vi "Teleop.vi"(10 "Match Info":T1={"Autonomous Elapsed Seconds"=0.0, "TeleOp Elapsed Seconds"=0.0, "Disabled Elapsed Seconds"=0.0, "Visited Autonomous"=FALSE, "Visited TeleOp"=FALSE, "Visited Disabled"=FALSE, "Autonomous Settings"={"Autonomous Style"=enum."Independent", "VI Refnum"=refnum}}, 11 "Call Context":T2) -> ()   [LabVIEW 2019]
doc: "This VI is called for each TeleOp packet received from the DS where the robot is not disabled. It is often used to read from the joysticks and update I/O or to update setpoints for timed control loops. It should complete and return within 20 milliseconds or it may miss DS packets."
uses:
  <vilib>/Rock Robotics/WPI/DriverStation/WPI_DriverStationDerivedRobotMode.ctl
  <vilib>/Rock Robotics/WPI/DriverStation/WPI_DriverStationMatch Info.ctl
  <vilib>/Rock Robotics/WPI/Utilities/WPI_GetSetVariantRefNum.vi
  Robot Global Data.vi
  fe9523e3-5247-4d02-ac38-c1c90a242367.vi
  0c9b3fa4-6825-40db-97e3-58cf3b513131.vi
  9558ccb8-c015-4717-8b16-c2a20c3b9826.vi
  ab49278a-ad98-44ea-a773-ace26d2c49d4.vi
panel:
  out "Axes":dbl[](array[numeric])
  in  "Color":string
  in  "ResetColorPos":bool
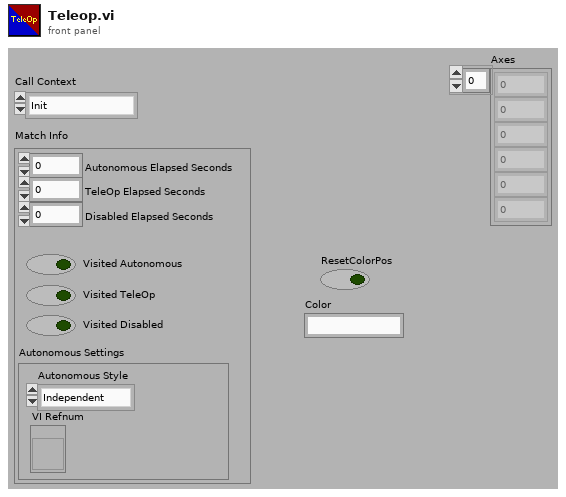
[diagram p1: front panel]
types:
  T1 = typedef "WPI_DriverStationMatch Info.ctl" = cluster{"Autonomous Elapsed Seconds":dbl, "TeleOp Elapsed Seconds":dbl, "Disabled Elapsed Seconds":dbl, "Visited Autonomous":bool, "Visited TeleOp":bool, "Visited Disabled":bool, "Autonomous Settings":cluster{"Autonomous Style":enum16{"Iterative", "Independent"}, "VI Refnum":refnum<vi>}}
  T2 = typedef "WPI_DriverStationDerivedRobotMode.ctl" = enum16{"Init", "Execute", "Stop"}
  T3 = typedef "WPI_JoystickDevRef.ctl" = cluster{"Device":T4}
  T4 = typedef "WPI_JoystickDeviceEnum.ctl" = enum16{"USB 0", "USB 1", "USB 2", "USB 3", "USB 4", "USB 5"}
  T5 = cluster{"ColorPosReached?":bool, "ColorRotButton":bool, "ColorRotReached?":bool, "ColorPosButton":bool}
  T6 = cluster{"Yaw":dbl, "Roll":dbl, "Pitch":dbl, "Heading":dbl, "Fused Heading":dbl}
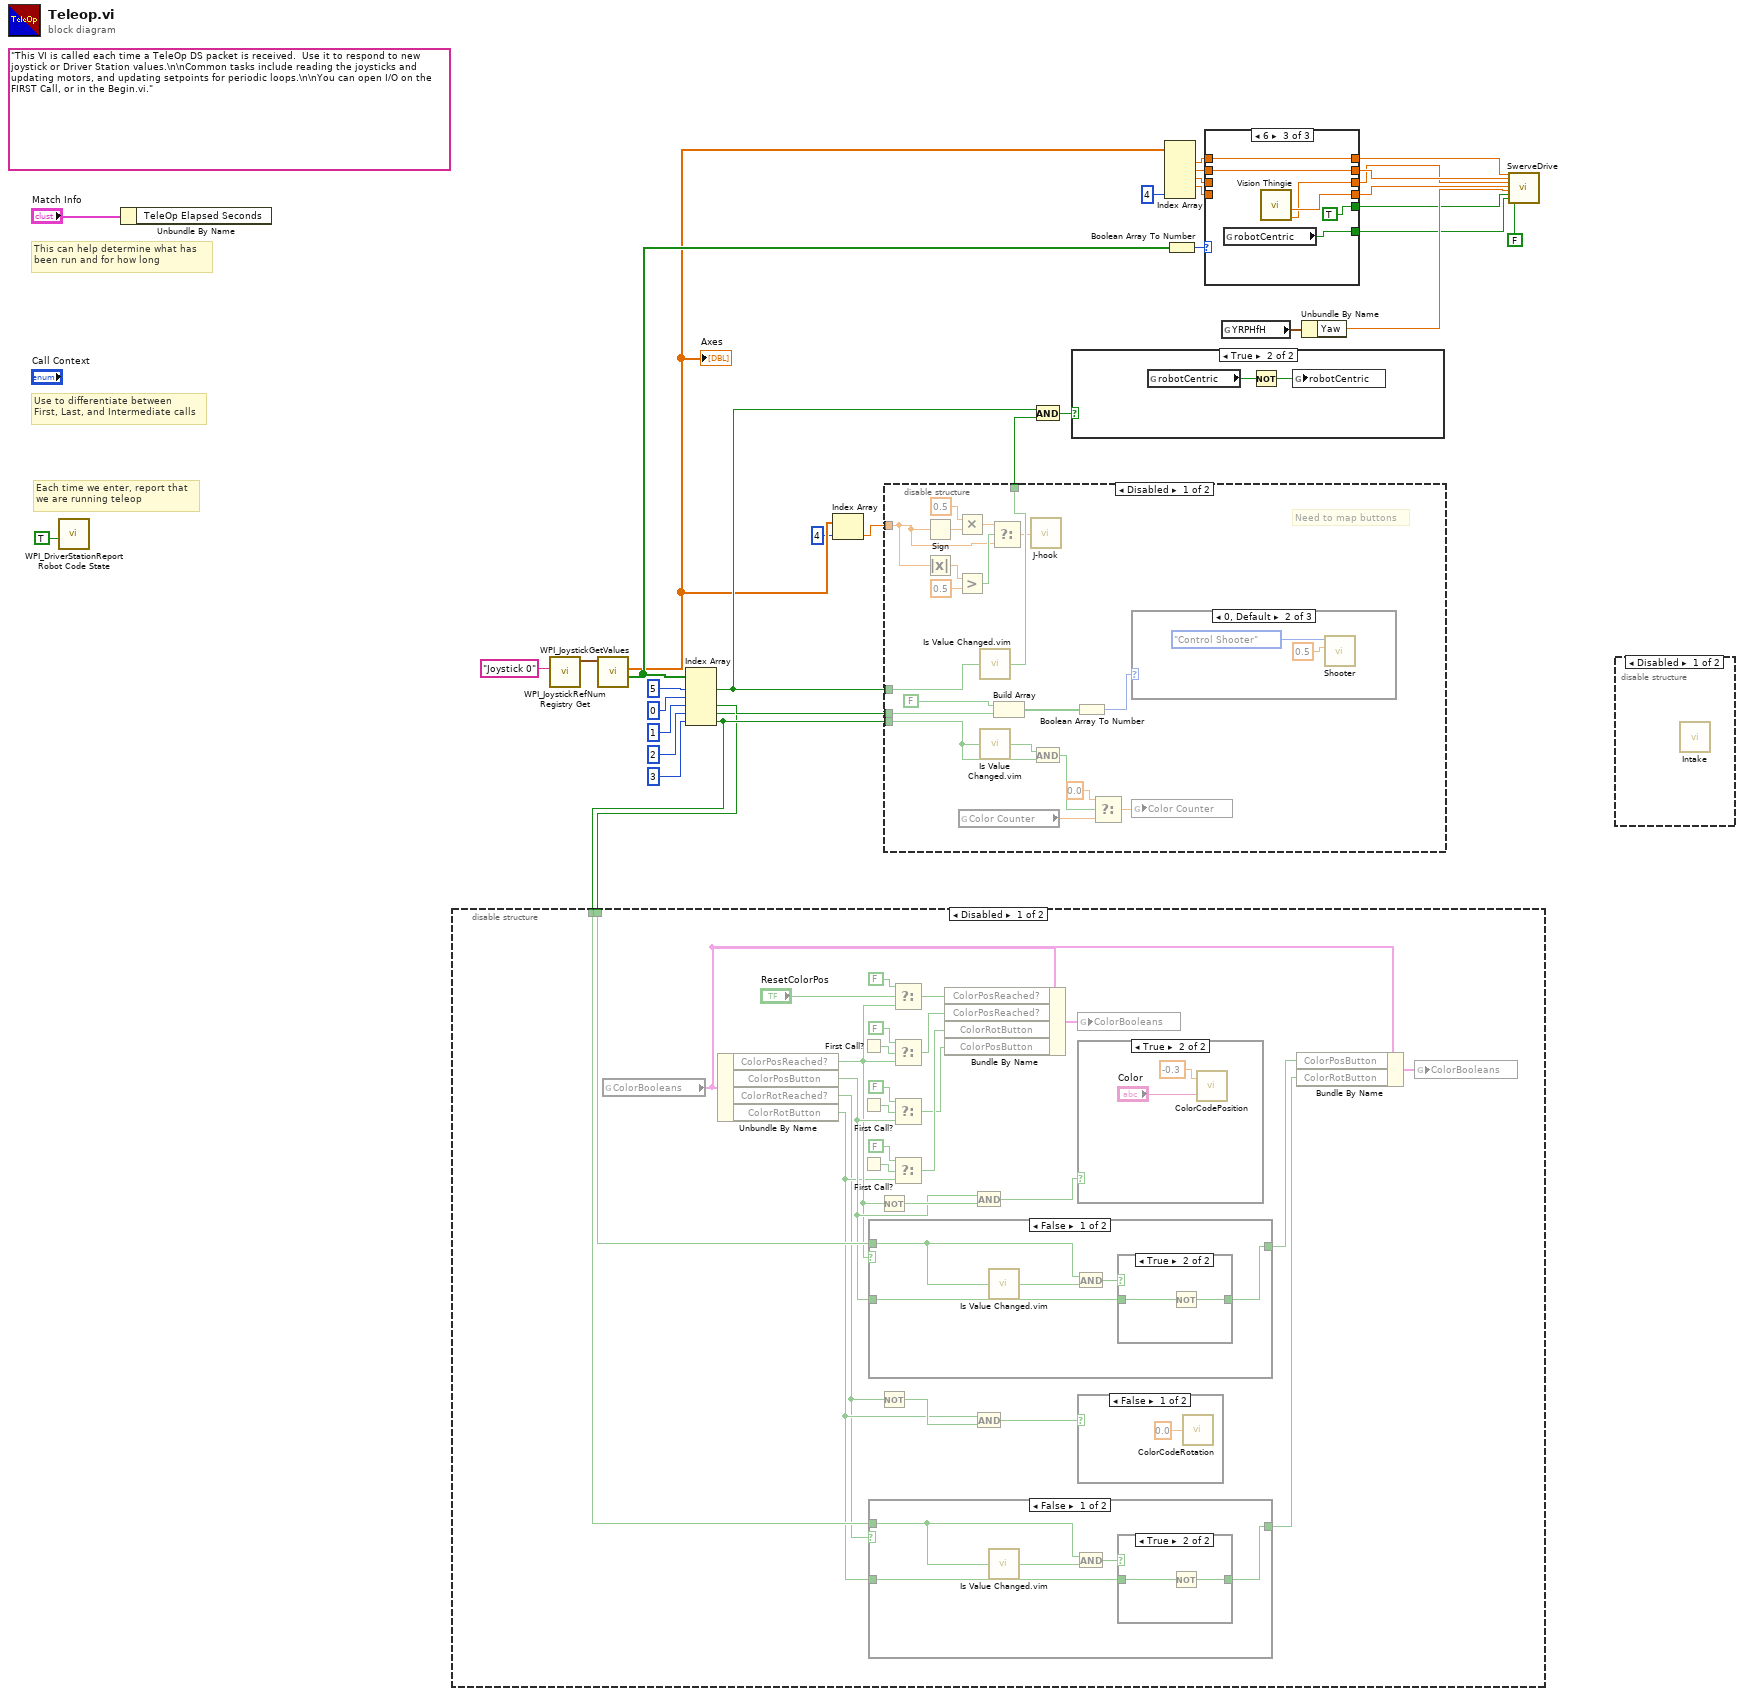
[diagram p0: block diagram]
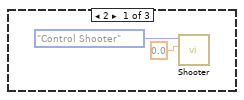
[diagram p3: hidden frame]
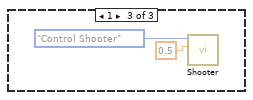
[diagram p4: hidden frame]
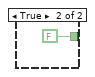
[diagram p7: hidden frame]
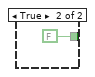
[diagram p9: hidden frame]
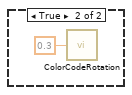
[diagram p10: hidden frame]
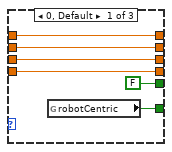
[diagram p13: hidden frame]
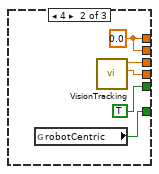
[diagram p14: hidden frame]
diagram:
  (unwired) "This VI is called each time a TeleOp DS packet is received.  Use it to respond to new joystick or Driver Station values.\n\nCommon tasks include reading the joysticks and updating motors, and updating setpoints for periodic loops.\n\nYou can open I/O on the FIRST Call, or in the Begin.vi."
  # "Each time we enter, report that\nwe are running teleop"
  # "Use to differentiate between\nFirst, Last, and Intermediate calls"
  # "This can help determine what has\nbeen run and for how long"
  n1 = call <vilib>:"WPI_DriverStationReport Robot Code State.vi"("TeleOp"=TRUE ("Autonomous")) -> ()  [unwired: 10 in, 1 out]
  n2 = Unbundle By Name("Match Info") -> ()  [unwired: 1 out]
  n3 = call <vilib>:"WPI_JoystickRefNum Registry Get.vi"("refnum name"="Joystick 0") -> ("JoystickDevRef"=w29:T3)  [unwired: 1 in, 9 out]
  n4 = call <vilib>:"WPI_JoystickGetValues.vi"("JoystickDevRef"=w29) -> ("Buttons"=w13:bool[], "Axes"=w3:dbl[])  [unwired: 6 in, 3 out]
  "Axes" <- w3
  n5 = Index Array(array=w13, index #1=5 ("index"), index #2=0 ("index"), index #3=1 ("index"), index #4=2 ("index"), index #5=3 ("index")) -> (element #1=w27:bool, element #3=w24:bool, element #4=w15:bool, element #5=w16:bool)  [unwired: 1 out]
  n6 = disable-structure shown="Disabled" {
    disable-tunnel: w16 -> [w61 _]
    disable-tunnel: w15 -> [w60 _]
    frame Disabled {
      n7 = global read "Robot Global Data.vi" "ColorBooleans"() -> (w37:T5)
      n8 = Unbundle By Name(w37) -> ("ColorPosReached?"=w46:bool, "ColorPosButton"=w47:bool, "ColorRotReached?"=w44:bool, "ColorRotButton"=w45:bool)
      n9 = First Call?() -> (First Call?: T/F=w50:bool)
      n10 = First Call?() -> (First Call?: T/F=w52:bool)
      n11 = First Call?() -> (First Call?: T/F=w55:bool)
      n12 = case shown="False" w46 {
        tunnel: w60 -> [w65 _]
        tunnel: w47 -> [w63 _]
        tunnel: [w62 FALSE ("ColorPosButton")] -> w35
        frame False {
          n13 = call "Is Value Changed.vim"("value"=w65) -> ("changed or first call?"=w66:bool)
          n14 = And(x=w65, y=w66) -> (x .and. y?=w64:bool)
          n15 = case shown="True" w64 {
            tunnel: w63 -> [w67 w69]
            tunnel: [w67 w68] -> w62
            frame False {
            }
            frame True {
              n16 = Not(x=w69) -> (.not. x?=w68:bool)
            }
          }
        }
        frame True {
        }
      }
      n17 = case shown="False" w44 {
        tunnel: w61 -> [w75 _]
        tunnel: w45 -> [w72 _]
        tunnel: [w71 FALSE ("ColorRotButton")] -> w36
        frame False {
          n18 = call "Is Value Changed.vim"("value"=w75) -> ("changed or first call?"=w74:bool)
          n19 = And(x=w75, y=w74) -> (x .and. y?=w73:bool)
          n20 = case shown="True" w73 {
            tunnel: w72 -> [w76 w78]
            tunnel: [w76 w77] -> w71
            frame False {
            }
            frame True {
              n21 = Not(x=w78) -> (.not. x?=w77:bool)
            }
          }
        }
        frame True {
        }
      }
      n22 = Not(x=w46) -> (.not. x?=w58:bool)
      n23 = Not(x=w44) -> (.not. x?=w57:bool)
      n24 = Select(t=FALSE, s="ResetColorPos", f=w46) -> (s? t:f=w42:bool)
      n25 = Select(t=FALSE, s=w50, f=w46) -> (s? t:f=w41:bool)
      n26 = Select(t=FALSE, s=w52, f=w47) -> (s? t:f=w39:bool)
      n27 = Select(t=FALSE, s=w55, f=w45) -> (s? t:f=w40:bool)
      n28 = Bundle By Name(cluster=w37, "ColorPosReached?"=w42, "ColorPosReached?"=w41, "ColorRotButton"=w40, "ColorPosButton"=w39) -> (w43:T5)
      n29 = And(x=w47, y=w58) -> (x .and. y?=w59:bool)
      n30 = And(x=w45, y=w57) -> (x .and. y?=w56:bool)
      n31 = global write "Robot Global Data.vi" "ColorBooleans"(w43) -> ()
      n32 = case shown="True" w59 {
        frame False {
        }
        frame True {
          n33 = call "ColorCodePosition.vi"("Color"="Color", "Output"=-0.3) -> ()  [unwired: 1 in]
        }
      }
      n34 = case shown="False" w56 {
        frame False {
          n35 = call "ColorCodeRotation.vi"("Output 2"=0.0) -> ()
        }
        frame True {
          n36 = call "ColorCodeRotation.vi"("Output 2"=0.3) -> ()
        }
      }
      n37 = Bundle By Name(cluster=w37, "ColorPosButton"=w35, "ColorRotButton"=w36) -> (w38:T5)
      n38 = global write "Robot Global Data.vi" "ColorBooleans"(w38) -> ()
    }
    frame Enabled {
    }
  }
  n39 = Index Array(array=w3, index=4) -> (element=w1:dbl)
  n40 = disable-structure shown="Disabled" {
    disable-tunnel: [w103 _] -> w31
    disable-tunnel: w27 -> [w102 _]
    disable-tunnel: w24 -> [w100 _]
    disable-tunnel: w16 -> [w98 _]
    disable-tunnel: w1 -> [w88 _]
    frame Disabled {
      # "Need to map buttons"
      n41 = Sign(1:w88) -> (0:w85:dbl)
      n42 = Absolute Value(x=w88) -> (abs(x)=w89:dbl)
      n43 = Multiply(x=0.5 ("t"), y=w85) -> (x*y=w86:dbl)
      n44 = Greater?(x=w89, y=0.5) -> (0:w90:bool)
      n45 = global read "Robot Global Data.vi" "Color Counter"() -> (w93:dbl)
      n46 = call "Is Value Changed.vim"("value"=w102) -> ("changed or first call?"=w103:bool)
      n47 = call "Is Value Changed.vim"("value"=w98) -> ("changed or first call?"=w96:bool)
      n48 = Select(t=w86, s=w90, f=w88) -> (s? t:f=w84:dbl)
      n49 = Build Array(FALSE ("element"), w100) -> (w101:bool[])
      n50 = call "J-hook.vi"("Output"=w84) -> ()
      n51 = And(x=w96, y=w98) -> (x .and. y?=w97:bool)
      n52 = Boolean Array To Number(Boolean array=w101) -> (number=w92:u32)
      n53 = Select(t=0.0, s=w97, f=w93) -> (s? t:f=w94:dbl)
      n54 = case shown="0, Default" w92 {
        frame 2 {
          n55 = call "Shooter.vi"("Shooter Output"=0.0, "Mode"=enum16{"Control Shooter", "Control Aim", "Open"}."Control Shooter") -> ()  [unwired: 10 in]
        }
        frame 0, Default {
          n56 = call "Shooter.vi"("Shooter Output"=0.5, "Mode"=enum16{"Control Shooter", "Control Aim", "Open"}."Control Shooter") -> ()  [unwired: 10 in]
        }
        frame 1 {
          n57 = call "Shooter.vi"("Shooter Output"=0.5, "Mode"=enum16{"Control Shooter", "Control Aim", "Open"}."Control Shooter") -> ()  [unwired: 10 in]
        }
      }
      n58 = global write "Robot Global Data.vi" "Color Counter"(w94) -> ()
    }
    frame Enabled {
    }
  }
  n59 = And(x=w27, y=w31) -> (x .and. y?=w30:bool)
  n60 = case shown="True" w30 {
    frame False {
    }
    frame True {
      n61 = global read "Robot Global Data.vi" "robotCentric"() -> (w111:bool)
      n62 = Not(x=w111) -> (.not. x?=w110:bool)
      n63 = global write "Robot Global Data.vi" "robotCentric"(w110) -> ()
    }
  }
  n64 = Index Array(array=w3, index #5=4 ("index")) -> (element #1=w11:dbl, element #2=w9:dbl, element #3=w7:dbl, element #4=w5:dbl)  [unwired: 4 in, 1 out]
  n65 = Boolean Array To Number(Boolean array=w13) -> (number=w14:u32)
  n66 = case shown="6" w14 {
    tunnel: [FALSE TRUE TRUE] -> w19
    tunnel: [w113 w121 w128] -> w18
    tunnel: [w117 w118 w125] -> w12
    tunnel: w11 -> [w117 _ w125]
    tunnel: [w116 w118 w124] -> w10
    tunnel: w9 -> [w116 _ w124]
    tunnel: [w115 w120 w123] -> w8
    tunnel: w7 -> [w115 _ _]
    tunnel: [w114 w119 w126] -> w6
    tunnel: w5 -> [w114 _ _]
    frame 0, Default {
      n67 = global read "Robot Global Data.vi" "robotCentric"() -> (w113:bool)
    }
    frame 4 {
      w118 = 0.0 ("upper limit")
      n68 = global read "Robot Global Data.vi" "robotCentric"() -> (w121:bool)
      n69 = call "VisionTracking.vi"() -> ("Rot z 2"=w119:dbl, "Rot z"=w120:dbl)  [unwired: 10 in]
    }
    frame 6 {
      n70 = global read "Robot Global Data.vi" "robotCentric"() -> (w128:bool)
      n71 = call "Vision Thingie.vi"() -> ("z"=w123:dbl, "z2"=w126:dbl)  [unwired: 8 in]
    }
  }
  n72 = global read "Robot Global Data.vi" "YRPHfH"() -> (w21:T6)
  n73 = Unbundle By Name(w21) -> ("Yaw"=w20:dbl)
  n74 = call "SwerveDrive.vi"("x"=w12, "y"=w10, "z"=w8, "z2"=w6, "Yaw"=w20, "Autonomous?"=w19, "Robot Centric?"=w18, "Slow"=FALSE) -> ()  [unwired: 20 in]
  n75 = disable-structure shown="Disabled" {
    frame Disabled {
      n76 = call "Intake.vi"() -> ()  [unwired: 12 in]
    }
    frame Enabled {
    }
  }
